vi "varying square wave.vi"() -> ()   [LabVIEW 2014]
panel:
  in  "ISI (frames)":i32
  in  "pulse duration (frames)":i32
  in  "Trials Per Power":i32
  in  "Power Array (uW/mm^2)":dbl[](array[numeric])
  in  "Min Power":dbl
  in  "Frames":i32
  in  "Transfer and Run Date Folder After Experiment":bool
  in  "SSH user name":string
  in  "SSH password":string
  in  "Wait before recording (s)":dbl
  in  "Tags":string
  in  "Start Recording":bool
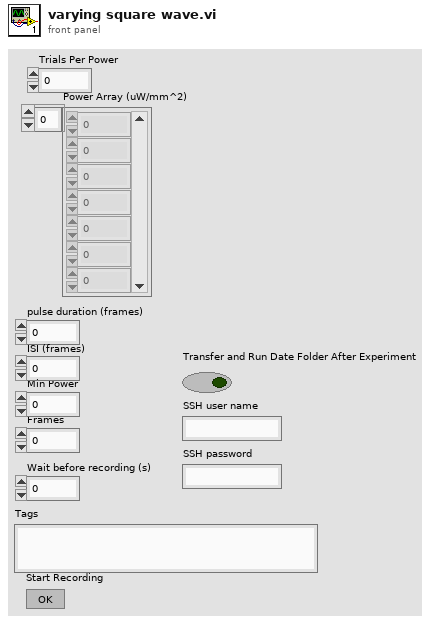
[diagram p1: front panel]
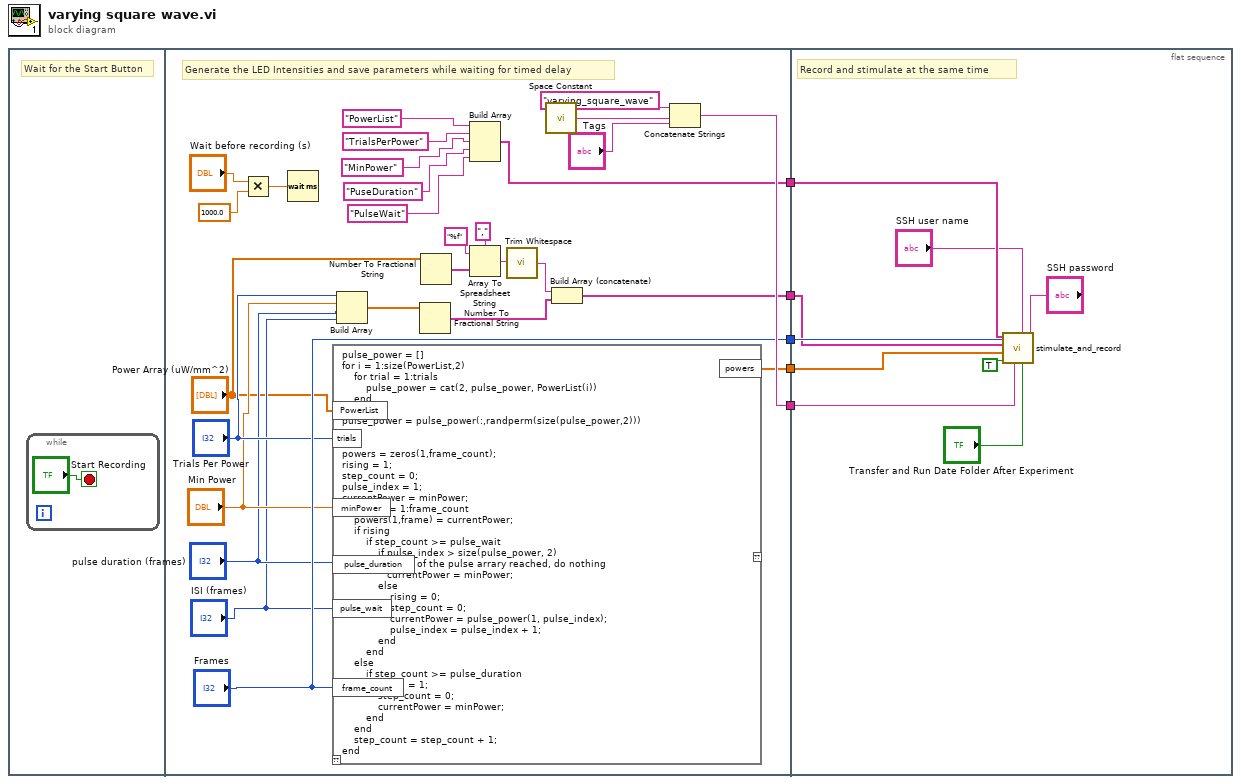
[diagram p0: block diagram]
diagram:
  n1 = flat-sequence {
    tunnel: [w31] -> w5
    tunnel: [w22] -> w4
    tunnel: [w21] -> w3
    tunnel: ["Frames"] -> w2
    tunnel: [w10] -> w1
    tunnel: w5 -> [w43]
    tunnel: w4 -> [w41]
    tunnel: w3 -> [w37]
    tunnel: w2 -> [w36]
    tunnel: w1 -> [w35]
    frame #0 {
      # "Wait for the Start Button"
      n2 = while {
        stop <- "Start Recording" stop-if-true
      }
    }
    frame #1 {
      # "Generate the LED Intensities and save parameters while waiting for timed delay"
      n3 = Multiply(x="Wait before recording (s)", y=1000.0) -> (x*y=w29:dbl)
      n4 = Wait (ms)(milliseconds to wait=w29) -> ()  [unwired: 1 out]
      n5 = script code="pulse_power = []\nfor i = 1:size(PowerList,2)\n    for trial = 1:trials\n        pulse_power = cat(2, pulse_power, PowerList(i))\n    end\nend\npulse_power = pulse_power(:,randperm(size(pulse_power,2)))\n\n\npowers = zeros(1,frame_count);\nrising = 1;\nstep_count = 0;\npulse_index = 1;\ncurrentPower = minPower;\nfor frame = 1:frame_count\n    powers(1,frame) = currentPower;\n    if rising\n        if step_count >= pulse_wait\n            if pulse_index > size(pulse_power, 2)\n               %end of the pulse arrary reached, do nothing\n               currentPower = minPower;\n            else\n                rising = 0;\n                step_count = 0;\n                currentPower = pulse_power(1, pulse_index);\n                pulse_index = pulse_index + 1;\n            end\n        end\n    else\n        if step_count >= pulse_duration\n            rising = 1;\n            step_count = 0;\n            currentPower = minPower;\n        end\n    end\n    step_count = step_count + 1;\nend"("pulse_duration"="pulse duration (frames)", "frame_count"="Frames", "trials"="Trials Per Power", "minPower"="Min Power", "PowerList"="Power Array (uW/mm^2)", "pulse_wait"="ISI (frames)") -> ("powers"=w21:dbl[])  [unwired: 1 in, 1 out]
      n6 = Build Array("Trials Per Power", "Min Power", "pulse duration (frames)", "ISI (frames)") -> (w14:dbl[])
      n7 = Number To Fractional String(number=w14) -> (F-format string=w11:string[])  [unwired: 3 in]
      n8 = Number To Fractional String(number="Power Array (uW/mm^2)") -> (F-format string=w13:string[])  [unwired: 3 in]
      n9 = Build Array("PowerList", "TrialsPerPower", "MinPower", "PuseDuration", "PulseWait") -> (w22:string[])
      n10 = Array To Spreadsheet String(delimiter (Tab)=",", array=w13, 3:"%f") -> (spreadsheet string=w8:string)
      n11 = call <vilib>:"Trim Whitespace.vi"("string"=w8) -> ("trimmed string"=w7:string)  [unwired: 1 in]
      n12 = call <vilib>:"Space Constant.vi"() -> ("String"=w33:string)
      n13 = Build Array (concatenate)(w7, w11) -> (w10:string[])
      n14 = Concatenate Strings("varying_square_wave", w33, "Tags") -> (w31:string)
    }
    frame #2 {
      # "Record and stimulate at the same time"
      n15 = call "stimulate_and_record.vi"("SSH password"="SSH password", "Transfer and Run Date Folder After Experiment"="Transfer and Run Date Folder After Experiment", "SSH user name"="SSH user name", "Tags"=w43, "Frames"=w36, "Convert Power to Voltage"=TRUE, "voltages/power"=w37, "parameters"=w35, "parameters headers"=w41) -> ()  [unwired: 3 in]
    }
  }
